vi "BI_VFFT measurement.vi"() -> ()   [LabVIEW 2023]
uses:
  <vilib>/Utility/file.llb/Write Delimited Spreadsheet (DBL).vi
panel:
  in  "Status":enum32{"Measurement Status"}(tab)
  in  "Comments":string="See the below notes for this measurement.SR785 Status:Fre Span 51200.000000\n Hz; Center Fre 25600.000000\n Hz; Points(0 for 101, 1 for 201, 2 for 401 3 for 801): 3\n; Start, End Fre: 0.000000\n, 51200.000000\nHz; Unit y: dBVpk\n;\n"
  out "Current FIeld":dbl=0.8
  out "Current Current":dbl=2.5
  out "error out":errorcluster
  in  "Response Control":enum32{"cRIO slow V", "SR785"}(tab)
  in  "scale":dbl=0.0001
  in  "Channel":string(combo)="AI0"
  in  "Average":i32=500
  out "FFT record time s":dbl=0.015625 caption="Delay Time (s)"
  in  "SR785 VISA":string="GPIB0::10::INSTR"
  in  "Display data":i32(ring) items=["Display A", "Display B"]
  in  "Center Hz":dbl=25000.0 format="%^.2e"
  in  "Span Hz":dbl=50000.0 format="%^.2e"
  in  "Resolution":i32(ring)=3 items=["100", "200", "400", "800"]
  in  "average num":i32=20
  out "CRIO pipe":T1={"DAQ_CMD_Writer endpoint"="DAQ_CMD_Writer", "DAQ_AI_Reader endpoint"="DAQ_AI_Reader", "vi reference"=refnum, "application reference"=refnum}
  in  "Excitation control":enum32{"B", "I"}(tab)
  in  "B Origin":dbl=-1.2 format="%#_13g"
  in  "B Radius":dbl=2.0 format="%#_13g"
  in  "B step":dbl=0.05 format="%#_13g"
  in  "B Ramp first":bool=TRUE
  in  "B Ramp type":string(combo)="Range"
  in  "Magnet Device Select":string(combo)="Elsa Magnet mT"
  in  "Field Rate mT per sec":dbl=0.1 format="%#_13g"
  in  "scale":dbl=1.0
  in  "I Origin":dbl format="%#_13g"
  in  "I step":dbl=0.01 format="%#_13g"
  in  "I Radius":dbl=2.5 format="%#_13g"
  in  "I Ramp first":bool=TRUE
  in  "I Ramp type":string(combo)="Range"
  in  "I Device Select":string(combo)="cRIO Slow"
  in  "AO Channel":string(combo)="AO0"
  in  "Book number":i32=685
  in  "parent data folder":path=path "C:/Users/gyue/Box/Guang Yue uiuc research box folder/data/Contour plot"
  # "This VI control measurements of multiple indenpent variable (Xs, such as B, I) and single channel data array (Yarray, FFT, V curve etc.)"
  # "Data structure: time-para.xml for all VI controls value, para.dat contains dimensions of data in form (x1 numbers, x2 numbers\\n y1 numbers, y2, numbers\\n y1 offset, y1 multipler\\n y2 offset, y2 multipler\\n ...), field.dat contains lines of independent variables at each measurement, data.dat contains measurment data line, one measurement per line or group of lines."
  # "Raw* scale=actual"
  # "Attation: The actuall frequency may different from set value, check the Comments control."
  # "value in uA x scale=raw"
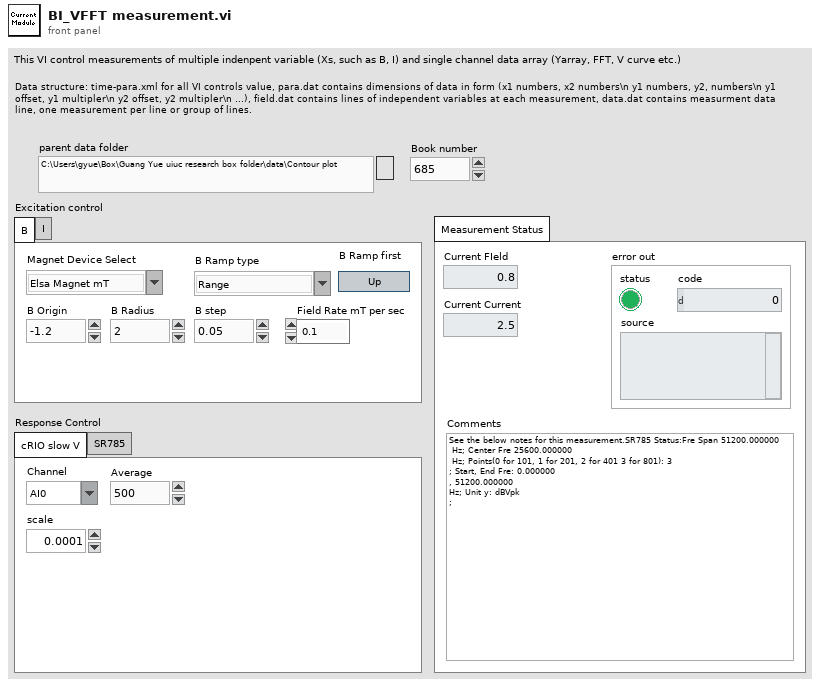
[diagram p1: front panel]
types:
  T1 = cluster{"DAQ_CMD_Writer endpoint":refnum<k21>, "DAQ_AI_Reader endpoint":refnum<k21>, "vi reference":refnum<vi>, "application reference":refnum<vi>}
  T2 = cluster{"AI0":dbl, "AI1":dbl, "AI2":dbl, "AI3":dbl}
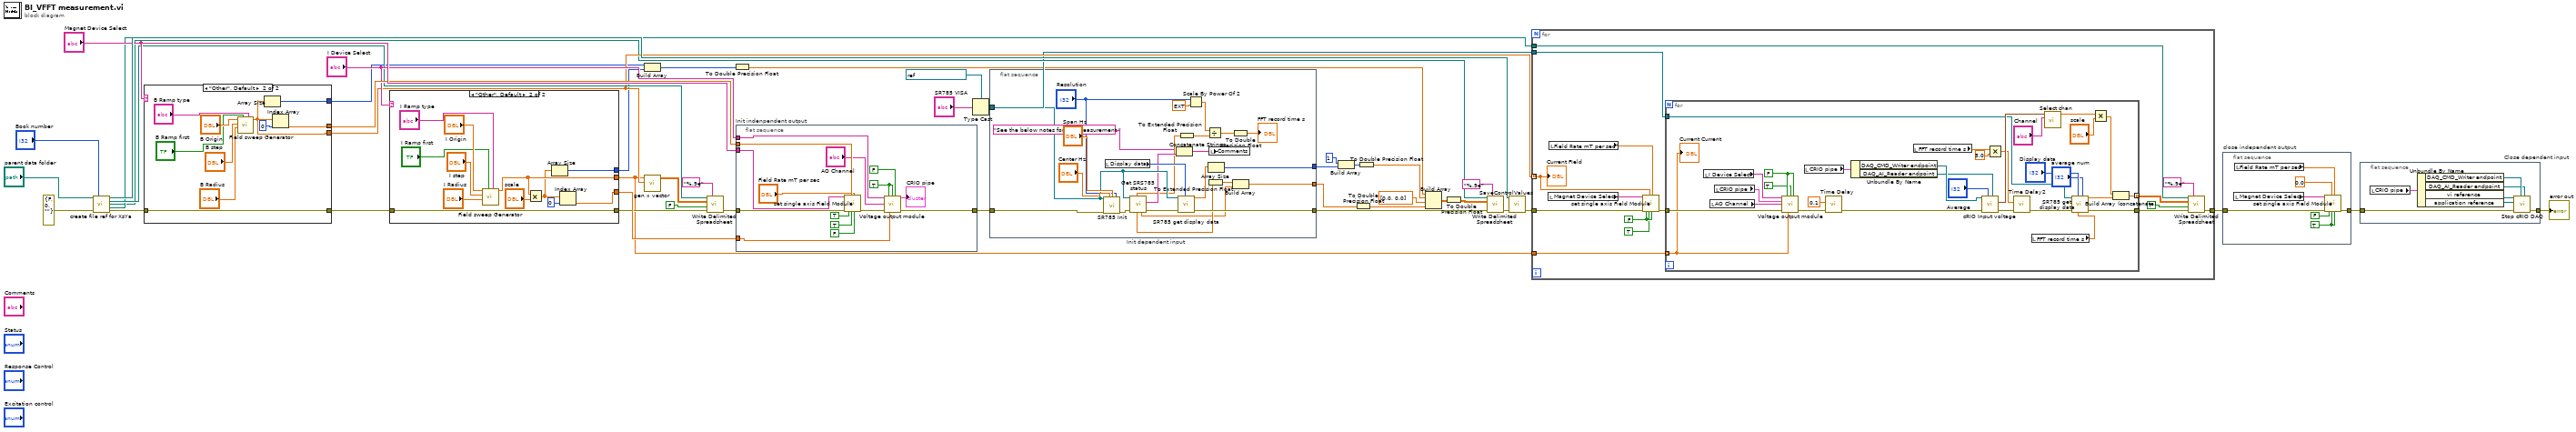
[diagram p0: block diagram]
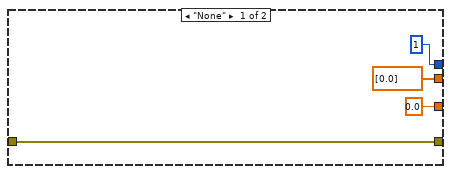
[diagram p2: hidden frame]
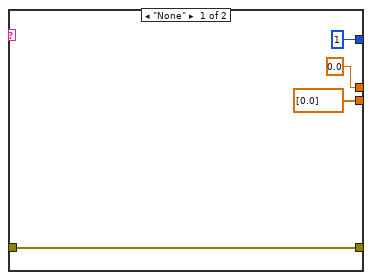
[diagram p3: hidden frame]
diagram:
  n1 = call "create file ref for XsYa.vi"("parent data folder"="parent data folder", "Book number"="Book number", "error in"=errorcluster {"status"=FALSE, "code"=0, "source"=""}) -> ("xml path"=w41:path, "field dat"=w32:path, "para dat"=w21:path, "data dat"=w26:path, "error out"=w8:errorcluster)  [unwired: 8 in]
  n2 = case shown="\"Other\", Default" "Magnet Device Select" {
    tunnel: [0.0 w52] -> w39
    tunnel: w8 -> [w47 w51]
    tunnel: [w47 w51] -> w36
    tunnel: [dbl[] [0.0] ("output array") w50] -> w29
    tunnel: [1 w49] -> w19
    frame "None" {
    }
    frame "Other", Default {
      n3 = call "Field sweep Generator.vi"("Ramp type"="B Ramp type", "Ramp up first T"="B Ramp first", "Field Radius"="B Radius", "Field step"="B step", "Field Origin"="B Origin") -> ("output array"=w50:dbl[])  [unwired: 6 in]
      n4 = Array Size(array=w50) -> (size(s)=w49:i32)
      n5 = Index Array(array=w50, index=0) -> (element=w52:dbl)
    }
  }
  n6 = case shown="\"Other\", Default" "I Device Select" {
    tunnel: [0.0 w68] -> w37
    tunnel: w36 -> [w61 w67]
    tunnel: [w61 w67] -> w35
    tunnel: [dbl[] [0.0] ("output array") w64] -> w28
    tunnel: [1 w65] -> w18
    frame "None" {
    }
    frame "Other", Default {
      n7 = call "Field sweep Generator.vi"("Ramp type"="I Ramp type", "Ramp up first T"="I Ramp first", "Field Radius"="I Radius", "Field step"="I step", "Field Origin"="I Origin") -> ("output array"=w64:dbl[])  [unwired: 6 in]
      n8 = Multiply(x=w64, y="scale") -> (x*y=w63:dbl[])
      n9 = Array Size(array=w63) -> (size(s)=w65:i32)
      n10 = Index Array(array=w63, index=0) -> (element=w68:dbl)
    }
  }
  n11 = Build Array(w19, w18) -> (w17:i32[])
  n12 = call "gen x vector.vi"("B"=w29, "I"=w28) -> ("Array"=w30:dbl[][])  [unwired: 9 in]
  n13 = call-poly <vilib>:"Write Delimited Spreadsheet.vi"("file path (dialog if empty)"=w32, "format (%.3f)"="%.9e", "2D data"=w30, "append to file? (new file:F)"=FALSE, "error in (no error)"=w35) -> ("error out"=w34:errorcluster)  [unwired: 9 in, 1 out]
  n14 = To Double Precision Float(number=w17) -> (double precision float=w5:dbl[])
  n15 = flat-sequence "Init indenpendent output" {
    tunnel: w34 -> [w77]
    tunnel: w39 -> [w86]
    tunnel: "Magnet Device Select" -> [w85]
    tunnel: "I Device Select" -> [w84]
    tunnel: w37 -> [w83]
    tunnel: [w76] -> w27
    frame #0 {
      w82 = TRUE ("Init")
      n16 = call "set single axis Field Module.vi"("Field Device Select"=w85, "error in (no error)"=w77, "Init"=TRUE, "Field Target mT or dBm"=w86, "Exec"=TRUE, "Field Rate mT per sec"="Field Rate mT per sec", "final"=FALSE) -> ("error out"=w80:errorcluster)  [unwired: 12 in]
      n17 = call "Voltage output module.vi"("Device Select"=w84, "Init"=w82, "Exec"=w82, "finish up"=FALSE, "AO Channel"="AO Channel", "Error In"=w80, "Voltage"=w83) -> ("current Control pipe"=→"CRIO pipe":T1, "Error out"=w76:errorcluster)  [unwired: 7 in]
    }
  }
  n18 = Type Cast(type=refnum<visa-resource-name> "GPIB0::10::INSTR" ("SR785 VISA"), x="SR785 VISA") -> (*(type *) &x=w12:refnum<visa-resource-name>)
  n19 = flat-sequence "Init dependent input" {
    tunnel: w27 -> [w110]
    tunnel: [w95] -> w9
    tunnel: w12 -> [w107]
    tunnel: [w111] -> w11
    tunnel: [w91] -> w2
    frame #0 {
      n20 = call "SR785 Init.vi"("VISA resource name"=w107, "Center (51.2E+3 Hz)"="Center Hz", "Span (102.4E+3 Hz)"="Span Hz", "Resolution (2: 400)"="Resolution", "error in (no error)"=w110) -> ("error out"=w97:errorcluster)  [unwired: 10 in]
      n21 = local read "Display data"() -> (w113:i32)
      n22 = call "Get SRS785 status.vi"("error in (no error)"=w97, "VISA resource name"=w107) -> ("error out"=w96:errorcluster, "concatenated string"=w106:string, "Fre multipler kHz"=w93:ext, "Fre start kHz"=w94:dbl, "Frequency Span"=w101:dbl)  [unwired: 3 in, 2 out]
      n23 = Concatenate Strings("See the below notes for this measurement." ("string"), w106) -> (w105:string)
      n24 = call "SR785 get display data.vi"("Display (0: Display A)"=w113, "error in (no error)"=w96, "VISA resource name"=w107) -> ("error out"=w95:errorcluster, "Waveform Graph"=w112:dbl[])  [unwired: 7 in]
      n25 = To Extended Precision Float(1:w101) -> (0:w100:ext)
      n26 = Scale By Power Of 2(n="Resolution", x=ext 100.0) -> (x*2^n=w102:ext)
      n27 = Divide(x=w102, y=w100) -> (x/y=w99:ext)
      n28 = Array Size(array=w112) -> (size(s)=w111:i32)
      n29 = To Extended Precision Float(1:w94) -> (0:w92:ext)
      n30 = local write "Comments"(w105) -> ()
      n31 = To Double Precision Float(number=w99) -> (double precision float=→"FFT record time s":dbl)
      n32 = Build Array(w92, w93) -> (w91:ext[])
    }
  }
  n33 = Build Array(1 ("element"), w11) -> (w15:i32[])
  n34 = To Double Precision Float(number=w2) -> (double precision float=w1:dbl[])
  n35 = To Double Precision Float(number=w15) -> (double precision float=w4:dbl[])
  n36 = Build Array(w5, w4, dbl[] [0.0, 0.0] ("element"), w1) -> (w14:dbl[][])
  n37 = To Double Precision Float(number=w14) -> (double precision float=w13:dbl[][])
  n38 = call-poly <vilib>:"Write Delimited Spreadsheet.vi"("file path (dialog if empty)"=w21, "format (%.3f)"="%.9e", "2D data"=w13, "error in (no error)"=w9) -> ("error out"=w7:errorcluster)  [unwired: 10 in, 1 out]
  n39 = call "SaveControlValues.vi"("XML File Path"=w41, "error in (no error)"=w7) -> ("error out"=w6:errorcluster)  [unwired: 8 in]
  n40 = for {
    tunnel: w29 -> [w124] mode=indexing
    tunnel: w6 -> [w128]
    tunnel: w28 -> [w122]
    tunnel: w12 -> [w120]
    tunnel: w26 -> [w119]
    tunnel: [w114] -> w10
    w126 = FALSE ("Init")
    n41 = local read "Magnet Device Select"() -> (w127:string)
    n42 = local read "Field Rate mT per sec"() -> (w123:dbl)
    n43 = call "set single axis Field Module.vi"("Field Device Select"=w127, "error in (no error)"=w128, "Init"=w126, "Field Target mT or dBm"=w124, "Exec"=TRUE, "Field Rate mT per sec"=w123, "final"=w126) -> ("error out"=w121:errorcluster)  [unwired: 12 in]
    n44 = for {
      tunnel: w122 -> [w153] mode=indexing
      tunnel: w121 -> [w159]
      tunnel: w120 -> [w141]
      tunnel: [w138] -> w117 mode=indexing
      tunnel: [w137] -> w116
      w156 = FALSE ("Init")
      n45 = local read "I Device Select"() -> (w158:string)
      n46 = local read "AO Channel"() -> (w157:string)
      n47 = local read "CRIO pipe"() -> (w154:T1)
      n48 = call "Voltage output module.vi"("Device Select"=w158, "Init"=w156, "Exec"=TRUE, "finish up"=w156, "Input Control pipe"=w154, "AO Channel"=w157, "Error In"=w159, "Voltage"=w153) -> ("Error out"=w152:errorcluster)  [unwired: 6 in, 1 out]
      n49 = local read "CRIO pipe"() -> (w149:T1)
      n50 = call "Time Delay"("error in (no error)"=w152, "Delay Time (s)"=0.1) -> ("error out"=w151:errorcluster)  [unwired: 9 in]
      n51 = Unbundle By Name(w149) -> ("DAQ_CMD_Writer endpoint"=w148:refnum<k21>, "DAQ_AI_Reader endpoint"=w147:refnum<k21>)
      n52 = local read "FFT record time s"() -> (w135:dbl)
      n53 = call "cRIO Input voltage.vi"("DAQ_AI_Reader endpoint"=w147, "Average"="Average", "error in (no error)"=w151, "DAQ_CMD_Writer endpoint"=w148) -> ("error out"=w145:errorcluster, "output cluster"=w144:T2)  [unwired: 5 in, 1 out]
      n54 = Multiply(x=w135, y=5.0) -> (x*y=w134:dbl)
      n55 = call "Time Delay2"("error in (no error)"=w145, "Delay Time (s)"=w134) -> ("error out"=w142:errorcluster)  [unwired: 9 in]
      n56 = local read "FFT record time s"() -> (w129:dbl)
      n57 = call "Select chan.vi"("Channel"="Channel", "output cluster"=w144) -> ("Output"=w139:dbl)  [unwired: 9 in]
      n58 = call "SR785 get display data.vi"("average num"="average num", "Delay Time (s)"=w129, "Display (0: Display A)"="Display data", "error in (no error)"=w142, "VISA resource name"=w141) -> ("error out"=w137:errorcluster, "Waveform Graph"=w136:dbl[])  [unwired: 5 in]
      n59 = Multiply(x=w139, y="scale") -> (x*y=w132:dbl)
      n60 = Build Array (concatenate)(w132, w136) -> (w138:dbl[])
      "Current Current" <- w153
    }
    n61 = call-poly <vilib>:"Write Delimited Spreadsheet.vi"("file path (dialog if empty)"=w119, "format (%.3f)"="%.9e", "2D data"=w117, "append to file? (new file:F)"=TRUE, "error in (no error)"=w116) -> ("error out"=w114:errorcluster)  [unwired: 9 in, 1 out]
    "Current FIeld" <- w124
  }
  n62 = flat-sequence "close independent output" {
    tunnel: w10 -> [w166]
    tunnel: [w165] -> w23
    frame #0 {
      w163 = TRUE ("Exec")
      n63 = local read "Magnet Device Select"() -> (w162:string)
      n64 = local read "Field Rate mT per sec"() -> (w160:dbl)
      n65 = call "set single axis Field Module.vi"("Field Device Select"=w162, "error in (no error)"=w166, "Init"=FALSE, "Field Target mT or dBm"=0.0 ("Field Target mT"), "Exec"=w163, "Field Rate mT per sec"=w160, "final"=w163) -> ("error out"=w165:errorcluster)  [unwired: 12 in]
    }
  }
  n66 = flat-sequence "Close dependent input" {
    tunnel: w23 -> [w173]
    tunnel: [w172] -> w22
    frame #0 {
      n67 = local read "CRIO pipe"() -> (w171:T1)
      n68 = Unbundle By Name(w171) -> ("DAQ_CMD_Writer endpoint"=w170:refnum<k21>, "DAQ_AI_Reader endpoint"=w169:refnum<k21>, "vi reference"=w168:refnum<vi>, "application reference"=w167:refnum<vi>)
      n69 = call "Stop cRIO DAQ.vi"("DAQ_AI_Reader endpoint"=w169, "DAQ_CMD_Writer endpoint"=w170, "error in (no error)"=w173, 10:w168, 11:w167) -> ("error out"=w172:errorcluster)  [unwired: 6 in]
    }
  }
  "error out" <- w22
